vi "lab2_sim_modem.vi"() -> ()   [LabVIEW 2014]
uses:
  <vilib>/addons/Modulation/Digital/General/MT Generate Bits (Galois, PN Order).vi
  <vilib>/addons/Modulation/Analog/support/mod_Set Error Source.vi
  <vilib>/addons/Modulation/Digital/Support/Common/Validators/mod_Generate Bits Validate.vi
  <vilib>/addons/Modulation/Digital/Support/Common/Validators/mod_AWGN Validate.vi
  <vilib>/addons/Modulation/Digital/Impairments/subVIs/mod_createSeeds.vi
  <vilib>/addons/Modulation/Digital/Support/Common/Validators/mod_Validate Samples Per Symbol.vi
  <vilib>/addons/Modulation/Analog/support/Validators/mod_Validate Complex Waveform.vi
  <vilib>/addons/Modulation/Analog/support/Validators/mod_WFErrorHandler.vi
  <vilib>/addons/Modulation/Digital/Support/Common/Validators/mod_Generate Filter Coefficients Validate.vi
  <vilib>/addons/Modulation/Digital/General/subVIs/mod_Generate Filter Coefficients.vi
  <vilib>/addons/Modulation/Digital/General/subVIs/mod_Generate Bits PN Sequence.vi
  <vilib>/addons/Modulation/Digital/General/MT Apply Pulse Shaping Filter (Generic).vi
  <vilib>/Analysis/1siggen.llb/Gaussian White Noise (obs 90).vi
  <vilib>/addons/Modulation/Digital/General/MT Apply Matched Filter (Generic).vi
  <vilib>/addons/Modulation/niDMT.lvlib
panel:
  out "ser/ber":dbl
  out "received symbols":u32
  out "error symbols":i32
  out "ser":dbl
  out "received bits":i32
  out "error bits":i32
  out "ber":dbl format="%#_5e"
  out "sync?":bool
  out "subarray":i16[](array[numeric])
  out "index map":u32[](array[numeric])
  out "output bit stream":i8[](array[numeric])
  in  "modulation":enum16{"PSK", "QAM"}(ring)
  in  "Gray code?":bool=TRUE
  out "size(s)":i32
  out "Received map":cdb[](graph)
  in  "Eb/N0 (10 dB)":dbl=10.0 format="%.2f"
  in  "samples per symbol":i32=16
  in  "filter parameter":dbl=0.5 format="%.2f"
  in  "filter length (symbols)":i32=8
  in  "pulse shaping filter (none)":T1(ring)=enum."Root Raised Cos"
  out "total bits":i32
  in  "total mod symbols":i32=2000 caption="total symbols"
  out "symbol map":cdb[](array[numeric])
  out "Transmitter map":cdb[](graph)
  in  "stop":bool
  in  "M-ARY":i32=4
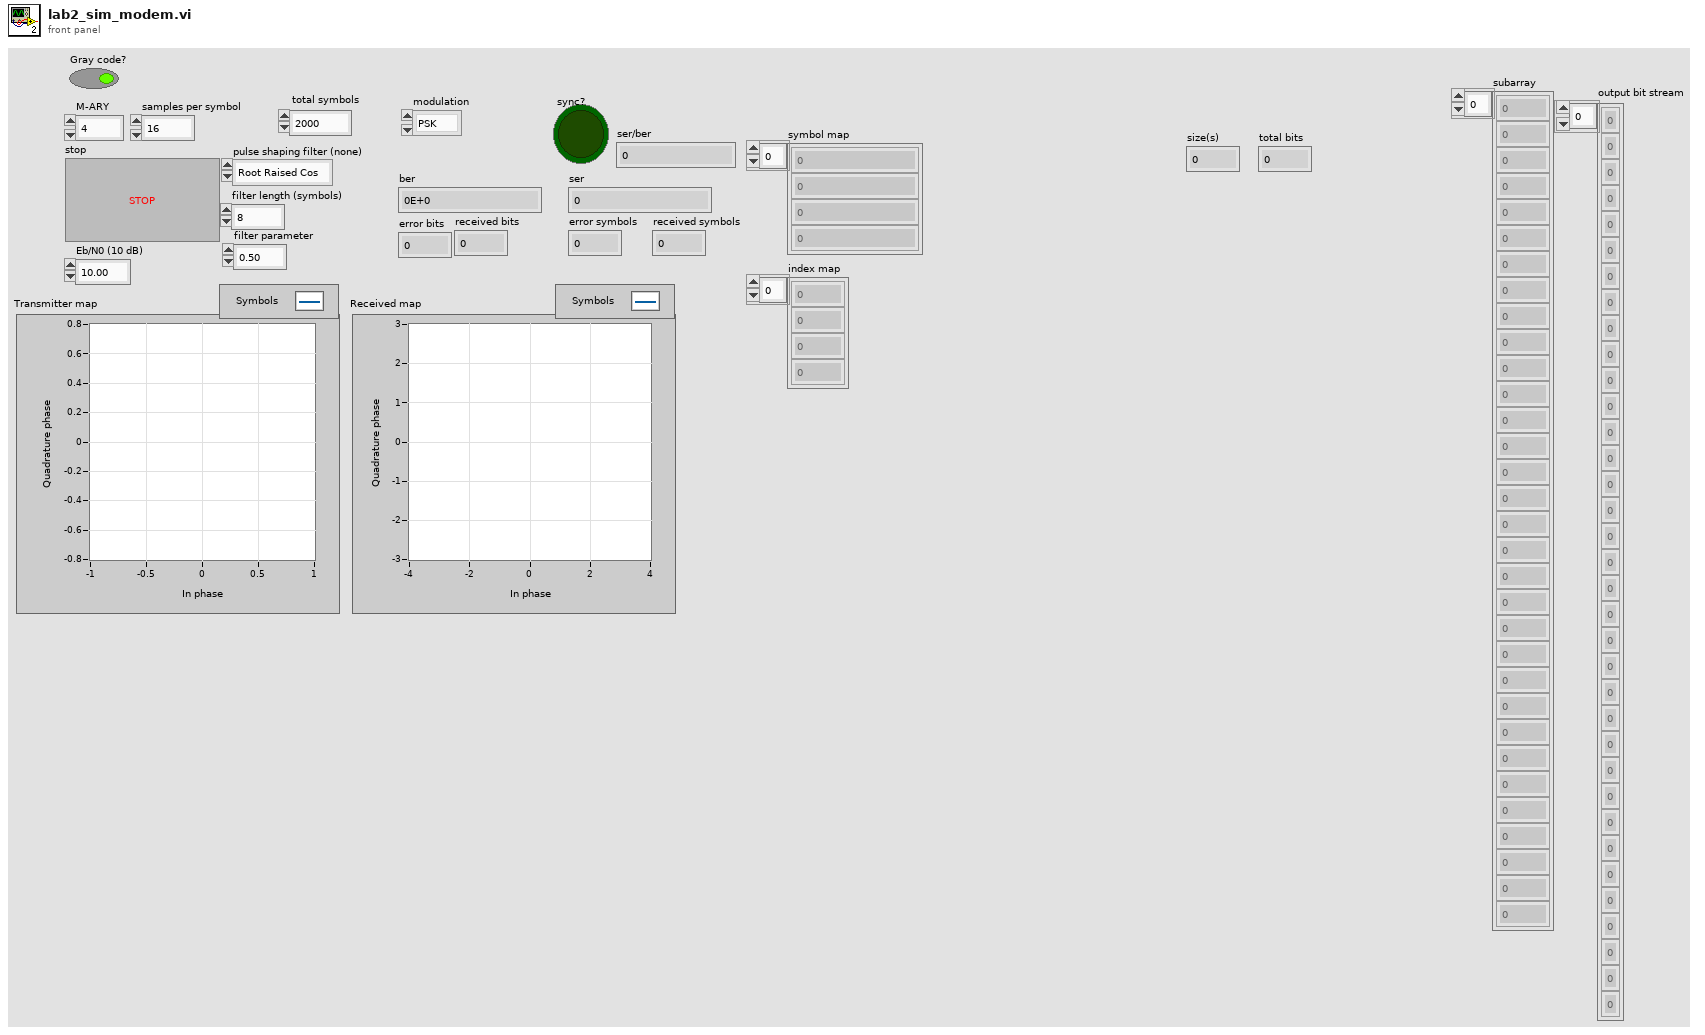
[diagram p1: front panel]
types:
  T1 = enum16{"none", "Raised Cosine", "Root Raised Cos", "Gaussian"}
  T2 = enum16{"FSK", "PSK", "QAM", "MSK", "PAM", "ASK", "CPM"}
  T3 = typedef "niAMT.lvlib/Complex Data Waveform.ctl" = cluster{"t0":dbl, "dt":dbl, "Y":cdb[]}
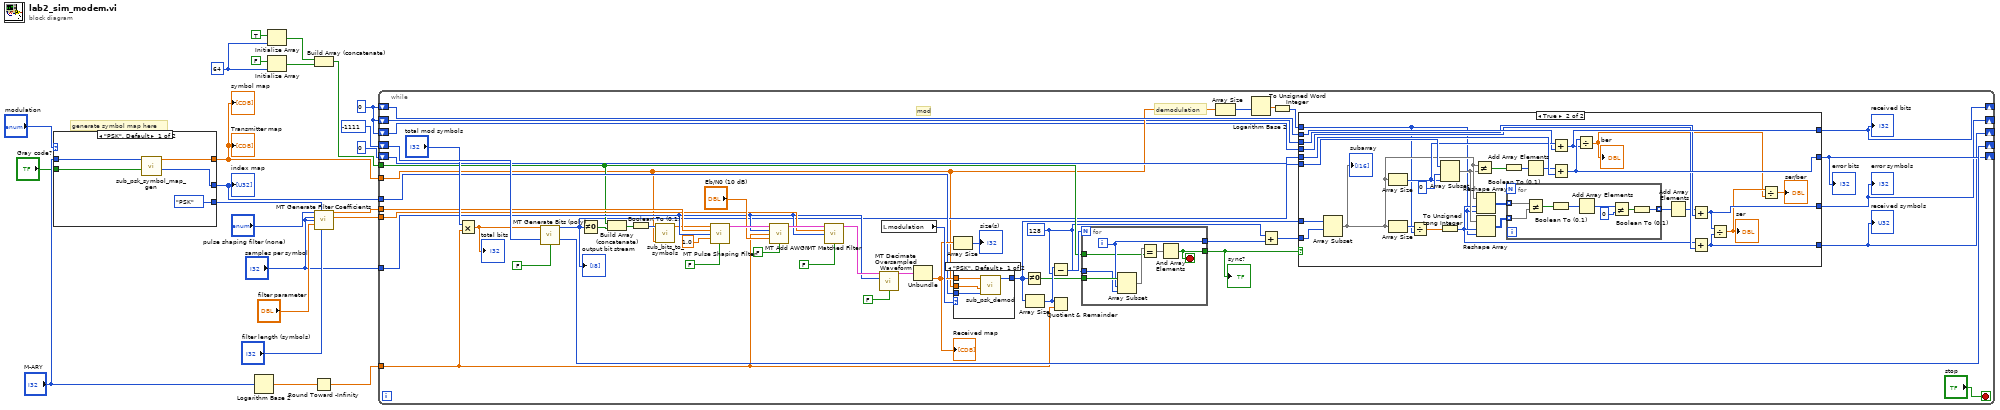
[diagram p0: block diagram]
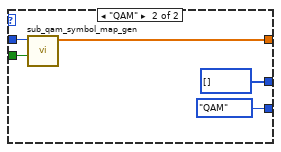
[diagram p2: hidden frame]
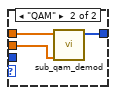
[diagram p4: hidden frame]
diagram:
  w1 = 0
  w3 = 64 ("dimension size")
  # "generate symbol map here"
  n1 = case shown="\"PSK\", Default" "modulation" {
    tunnel: "M-ARY" -> [w27 w33]
    tunnel: "Gray code?" -> [w28 w32]
    tunnel: [w26 w31] -> w11
    tunnel: [T2."PSK" ("modulation type") T2."QAM" ("modulation type")] -> w10
    tunnel: [w24 u32[] [] ("index map")] -> w9
    frame "PSK", Default {
      n2 = call "sub_psk_symbol_map_gen.vi"("Gray code?"=w28, "M-PSK"=w27) -> ("index map"=w24:u32[], "symbol map"=w26:cdb[])  [unwired: 8 in]
    }
    frame "QAM" {
      n3 = call "sub_qam_symbol_map_gen.vi"("Gray code?"=w32, "M-QAM"=w33) -> ("symbol map"=w31:cdb[])  [unwired: 9 in]
    }
  }
  "Transmitter map" <- w11
  "symbol map" <- w11
  "index map" <- w9
  n4 = Logarithm Base 2(1:"M-ARY") -> (0:w23:dbl)
  n5 = Initialize Array(TRUE, w3) -> (w8:bool[])
  n6 = Initialize Array(FALSE, w3) -> (w7:bool[])
  n7 = Round Toward -Infinity(1:w23) -> (0:w16:dbl)
  n8 = Build Array (concatenate)(w8, w7) -> (w4:bool[])
  n9 = call <vilib>:"MT Generate Filter Coefficients.vi"("pulse shaping filter (none)"="pulse shaping filter (none)", "modulation type"=w10, "pulse shaping samples per symbol (16)"="samples per symbol", "matched samples per symbol (16)"="samples per symbol", "filter parameter"="filter parameter", "filter length (symbols)"="filter length (symbols)") -> ("pulse shaping filter coefficients"=w18:dbl[], "matched filter coefficients"=w15:dbl[])  [unwired: 7 in, 1 out]
  n10 = while {
    tunnel: w11 -> [w41]
    shift-right: [w81] -> _
    shift-left: -1111 ("seed out") -> [w82]
    tunnel: w18 -> [w78]
    tunnel: "samples per symbol" -> [w68]
    tunnel: w16 -> [w62]
    tunnel: w15 -> [w70]
    tunnel: w9 -> [w63]
    tunnel: w4 -> [w57]
    shift-right: [w48] -> _
    shift-left: 0 -> [w49]
    shift-right: [w46] -> _
    shift-left: w1 -> [w47]
    shift-right: [w38] -> _
    shift-left: w1 -> [w40]
    shift-right: [w37] -> _
    shift-left: w1 -> [w39]
    stop <- "stop" stop-if-true
    w51 = 128
    # "demodulation"
    # "mod"
    n11 = Multiply(x="total mod symbols", y=w62) -> (x*y=w80:dbl)
    "total bits" <- w80
    n12 = call-poly <vilib>:"MT Generate Bits (poly).vi"("total bits (128)"=w80, "seed in (0xD6BF7DF2)"=w82, "reset? (T)"=FALSE) -> ("output bit stream"=w50:i8[], "seed out"=w81:i32)  [unwired: 10 in, 1 out]
    "output bit stream" <- w50
    n13 = Not Equal To 0?(x=w50) -> (x != 0?=w60:bool[])
    n14 = Build Array (concatenate)(w57, w60) -> (w44:bool[])
    n15 = Boolean To (0,1)(Boolean=w44) -> (0, 1=w43:i16[])
    n16 = call "sub_bits_to_symbols.vi"("symbol map"=w41, "bits"=w43) -> ("symbols"=w42:cdb[])  [unwired: 9 in]
    n17 = call-poly <vilib>:"MT Pulse Shaping Filter.vi"("symbols"=w42, "pulse shaping filter coefficients"=w78, "samples per symbol (16)"=w68, "symbol rate (Hz)"=1.0, "reset? (T)"=FALSE) -> ("output complex waveform"=w74:T3)  [unwired: 9 in, 1 out]
    n18 = call <vilib>:"MT Add AWGN.vi"("input complex waveform"=w74, "samples per symbol (16)"=w68, "bits per symbol (1)"=w62, "Eb/N0 (10 dB)"="Eb/N0 (10 dB)", "reset? (T)"=FALSE) -> ("output complex waveform"=w71:T3)  [unwired: 8 in, 2 out]
    n19 = call-poly <vilib>:"MT Matched Filter.vi"("input complex waveform"=w71, "matched filter coefficients"=w70, "samples per symbol (16)"=w68, "reset? (T)"=FALSE) -> ("output complex waveform"=w69:T3)  [unwired: 10 in, 1 out]
    n20 = call <vilib>:"MT Decimate Oversampled Waveform.vi"("input complex waveform"=w69, "decimation factor"=w68, "reset? (T)"=FALSE) -> ("output complex waveform"=w67:T3)  [unwired: 11 in, 1 out]
    n21 = local read "modulation"() -> (w65:enum16{"PSK", "QAM"})
    n22 = Unbundle(w67) -> ("Y"=w64:cdb[])  [unwired: 2 out]
    "Received map" <- w64
    n23 = Array Size(array=w64) -> (size(s)=→"size(s)":i32)
    n24 = case shown="\"PSK\", Default" w65 {
      tunnel: w64 -> [w135 w137]
      tunnel: w41 -> [w134 w138]
      tunnel: w63 -> [w133 _]
      tunnel: [w132 w136] -> w54
      frame "PSK", Default {
        n25 = call "sub_psk_demod.vi"("index map"=w133, "symbol map"=w134, "symbol"=w135) -> ("bitstream"=w132:i16[])  [unwired: 8 in]
      }
      frame "QAM" {
        n26 = call "sub_qam_demod.vi"("symbol map"=w138, "symbol"=w137) -> ("bitstream"=w136:i16[])  [unwired: 9 in]
      }
    }
    n27 = Not Equal To 0?(x=w54) -> (x != 0?=w55:bool[])
    n28 = Array Size(array=w54) -> (size(s)=w59:i32)
    n29 = Subtract(x=w59, y=w51) -> (x-y=w58:i32)
    n30 = Quotient & Remainder(x=w59, y=w62) -> ()  [unwired: 2 out]
    n31 = for {
      N: w58 -> [_]
      tunnel: w55 -> [w131]
      tunnel: [w130] -> w53
      tunnel: w51 -> [w129]
      tunnel: w57 -> [w127]
      tunnel: [w125] -> w56
      i -> [w130]
      stop <- w125 stop-if-true
      n32 = Array Subset(array=w131, index=w130, length=w129) -> (w128:bool[])
      n33 = Equal?(x=w128, y=w127) -> (x = y?=w126:bool[])
      n34 = And Array Elements(Boolean array=w126) -> (logical AND=w125:bool)
    }
    "sync?" <- w56
    n35 = Array Size(array=w41) -> (size(s)=w36:i32)
    n36 = Logarithm Base 2(1:w36) -> (0:w35:dbl)
    n37 = Add(x=w51, y=w53) -> (x+y=w52:i32)
    n38 = To Unsigned Word Integer(number=w35) -> (unsigned 16bit integer=w34:u16)
    n39 = case shown="True" w56 {
      tunnel: w54 -> [_ w116]
      tunnel: w52 -> [_ w115]
      tunnel: w50 -> [_ w113]
      tunnel: w49 -> [w87 w110]
      tunnel: [w87 w108] -> w48
      tunnel: w47 -> [w86 w106]
      tunnel: [w86 w105] -> w46
      tunnel: w40 -> [w85 w95]
      tunnel: w39 -> [w84 w97]
      tunnel: [w84 w93] -> w37
      tunnel: [w85 w92] -> w38
      tunnel: w34 -> [_ w91]
      frame False {
      }
      frame True {
        n40 = Array Subset(array=w116, index=w115) -> (w102:i16[])  [unwired: 1 in]
        "subarray" <- w102
        n41 = Array Size(array=w102) -> (size(s)=w107:i32)
        n42 = Array Size(array=w102) -> (size(s)=w104:i32)
        n43 = Divide(x=w104, y=w91) -> (x/y=w103:dbl)
        n44 = Array Subset(array=w113, index=0, length=w107) -> (w101:i8[])
        n45 = To Unsigned Long Integer(number=w103) -> (unsigned 32bit integer=w96:u32)
        n46 = Not Equal?(x=w102, y=w101) -> (x != y?=w112:bool[])
        n47 = Reshape Array(w102, w96, w91) -> (w100:i16[][])
        n48 = Reshape Array(w101, w96, w91) -> (w99:i8[][])
        n49 = Boolean To (0,1)(Boolean=w112) -> (0, 1=w111:i16[])
        n50 = for {
          tunnel: w100 -> [w124] mode=indexing
          tunnel: w99 -> [w123] mode=indexing
          tunnel: [w117] -> w98 mode=indexing
          n51 = Not Equal?(x=w124, y=w123) -> (x != y?=w122:bool[])
          n52 = Boolean To (0,1)(Boolean=w122) -> (0, 1=w121:i16[])
          n53 = Add Array Elements(numeric array=w121) -> (sum=w120:i16)
          n54 = Not Equal?(x=w120, y=0) -> (x != y?=w118:bool)
          n55 = Boolean To (0,1)(Boolean=w118) -> (0, 1=w117:i16)
        }
        n56 = Add Array Elements(numeric array=w111) -> (sum=w109:i16)
        n57 = Add(x=w107, y=w106) -> (x+y=w105:i32)
        n58 = Add(x=w109, y=w110) -> (x+y=w108:i32)
        n59 = Divide(x=w108, y=w105) -> (x/y=w89:dbl)
        "ber" <- w89
        n60 = Add Array Elements(numeric array=w98) -> (sum=w94:i16)
        n61 = Add(x=w94, y=w95) -> (x+y=w92:i32)
        n62 = Add(x=w96, y=w97) -> (x+y=w93:u32)
        n63 = Divide(x=w92, y=w93) -> (x/y=w90:dbl)
        "ser" <- w90
        n64 = Divide(x=w90, y=w89) -> (x/y=→"ser/ber":dbl)
      }
    }
    "error bits" <- w48
    "received bits" <- w46
    "error symbols" <- w38
    "received symbols" <- w37
  }
